vi "Get Firmware Head.vi"(0 "COM Port In":refnum<visa-resource-name>, 1 "error in":errorcluster) -> (2 "COM Port out":refnum<visa-resource-name>, 3 "Firmware Head":string, 4 "OK":bool, 5 "error out":errorcluster)   [LabVIEW 2013]
doc: "This command may be used to get some additional information about the connected laser\nhead.\nThe syntax is equal to the “?GFw” command."
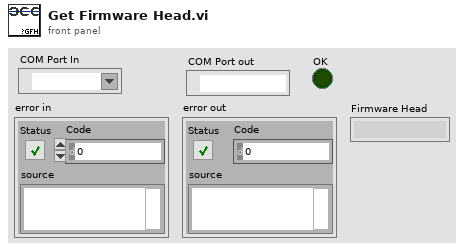
[diagram p1: front panel]
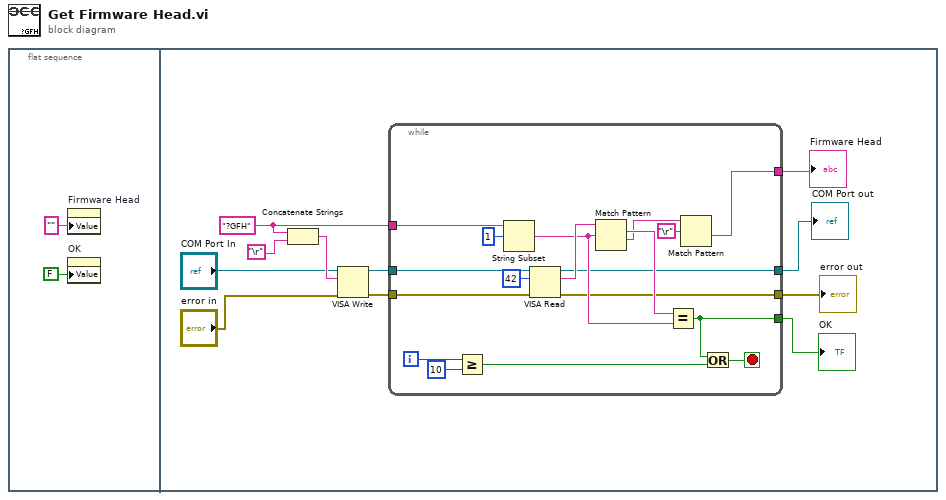
[diagram p0: block diagram]
diagram:
  n1 = flat-sequence {
    frame #0 {
      n2 = property on="Firmware Head" class="Str"("Value"="" ("Firmware Head")) -> ()  [unwired: 2 in, 2 out]
      n3 = property on="OK" class="Bool. (strikt)"("Value"=FALSE ("OK")) -> ()  [unwired: 2 in, 2 out]
    }
    frame #1 {
      w6 = "?GFH" ("Schreibpuffer")
      n4 = Concatenate Strings(w6, "\r") -> (w10:string)
      n5 = VISA Write(VISA resource name="COM Port In", write buffer=w10, error in (no error)="error in") -> (VISA resource name out=w5:refnum<visa-resource-name>, error out=w4:errorcluster)  [unwired: 1 out]
      n6 = while {
        tunnel: [w25] -> w13
        tunnel: [w24] -> w12
        tunnel: [w23] -> w11
        tunnel: w6 -> [w18]
        tunnel: w5 -> [w15]
        tunnel: w4 -> [w17]
        tunnel: [w16] -> w3
        i -> [w22]
        stop <- w19 stop-if-true
        n7 = Greater Or Equal?(x=w22, y=10) -> (x >= y?=w20:bool)
        n8 = String Subset(string=w18, offset (0)=1 ("Offset (0)")) -> (substring=w26:string)  [unwired: 1 in]
        n9 = VISA Read(VISA resource name=w15, byte count=u32 42 ("Byte-Anzahl"), error in (no error)=w17) -> (VISA resource name out=w24:refnum<visa-resource-name>, read buffer=w30:string, error out=w25:errorcluster)  [unwired: 1 out]
        n10 = Match Pattern(string=w30, regular expression=w26) -> (match substring=w29:string, after substring=w28:string)  [unwired: 1 in, 2 out]
        n11 = Equal?(x=w29, y=w26) -> (x = y?=w16:bool)
        n12 = Match Pattern(string=w28, regular expression="\r" ("Nach String/Zeichen suchen (-)")) -> (after substring=w23:string)  [unwired: 1 in, 3 out]
        n13 = Or(x=w16, y=w20) -> (x .or. y?=w19:bool)
      }
      "error out" <- w13
      "COM Port out" <- w12
      "Firmware Head" <- w11
      "OK" <- w3
    }
  }
